vi "Konversi_While Loop.vi"() -> ()   [LabVIEW 2020]
panel:
  in  "Celcius":dbl(slide) scale=0.0..100.0
  out "Reamur":dbl(slide) scale=0.0..80.0
  out "Kelvin":dbl(slide) scale=273.0..373.0
  out "Fahrenheit":dbl(slide) scale=32.0..212.0
  in  "stop 2":bool
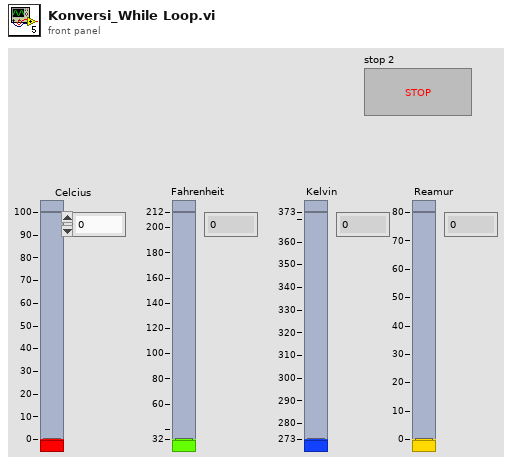
[diagram p1: front panel]
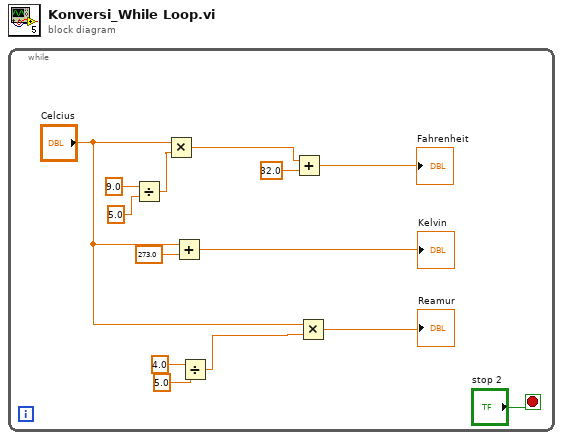
[diagram p0: block diagram]
diagram:
  n1 = while {
    stop <- "stop 2" stop-if-true
    n2 = Divide(x=9.0, y=5.0) -> (x/y=w13:dbl)
    n3 = Multiply(x="Celcius", y=w13) -> (x*y=w10:dbl)
    n4 = Add(x="Celcius", y=273.0) -> (x+y=→"Kelvin":dbl)
    n5 = Divide(x=4.0, y=5.0) -> (x/y=w4:dbl)
    n6 = Add(x=w10, y=32.0) -> (x+y=→"Fahrenheit":dbl)
    n7 = Multiply(x="Celcius", y=w4) -> (x*y=→"Reamur":dbl)
  }
